vi "Read Configuration with Unknown Modules.vi"() -> ()   [LabVIEW 2017]
uses:
  Types/Module Channel Settings.ctl
  <vilib>/addons/VeriStand Custom Device Scripting APIs/Scan Engine/Modules/Mode Classes/Controls/counter driven output channel settings.ctl
  <vilib>/addons/VeriStand Custom Device Scripting APIs/Scan Engine/Modules/Channel Classes/Counter Driven Output Channel/Counter Driven State.ctl
  <vilib>/addons/VeriStand Custom Device Scripting APIs/Scan Engine/Modules/Mode Classes/Controls/pwm channel settings.ctl
  <vilib>/addons/VeriStand Custom Device Scripting APIs/Scan Engine/Modules/Channel Classes/PWM Output Channel/Frequency.ctl
  <vilib>/addons/VeriStand Custom Device Scripting APIs/Scan Engine/Modules/NI 9474/NI 9474.lvclass
  f6bbfe02-b953-4ef2-a52c-5a4fac125821.vi
  <vilib>/addons/VeriStand Custom Device Scripting APIs/Scan Engine/Scan Engine Dependencies.llb/Set Error.vi
  <vilib>/Utility/error.llb/Clear Errors.vi
  <vilib>/addons/VeriStand Custom Device Scripting APIs/Scan Engine/Utility/Convert Slot Configuration to 9212.vi
  <vilib>/addons/VeriStand Custom Device Scripting APIs/Scan Engine/Utility/Convert Slot Configuration to 9213.vi
  <vilib>/addons/VeriStand Custom Device Scripting APIs/Scan Engine/Modules.lvlibp/SD Module/SD Module.lvclass
  C:/Program Files (x86)/National Instruments/LabVIEW 2017/vi.lib/addons/VeriStand Custom Device Scripting APIs/Scan Engine/Modules.lvlibp/RSI Module/RSI Module.lvclass
  <vilib>/addons/VeriStand Custom Device Scripting APIs/Scan Engine/Modules/NI 9212/NI 9212.lvclass
  C:/Program Files (x86)/National Instruments/LabVIEW 2017/vi.lib/addons/VeriStand Custom Device Scripting APIs/Scan Engine/Modules/Module/Module.lvclass
  <vilib>/addons/VeriStand Custom Device Scripting APIs/Scan Engine/Modules/NI 9213/NI 9213.lvclass
  <vilib>/addons/VeriStand Custom Device Scripting APIs/Scan Engine/Modules/NI 9224/NI 9224.lvclass
  <vilib>/addons/VeriStand Custom Device Scripting APIs/Scan Engine/Modules/NI 9228/NI 9228.lvclass
  <vilib>/addons/VeriStand Custom Device Scripting APIs/Scan Engine/Modules.lvlibp/RSI Module/Read Module Page Property.vi
  <vilib>/addons/VeriStand Custom Device Scripting APIs/Scan Engine/Modules.lvlibp/RSI Module/Read Model.vi
  <vilib>/addons/VeriStand Custom Device Scripting APIs/Scan Engine/Utility/Convert Module Model to Module Class.vi
  <vilib>/addons/VeriStand Custom Device Scripting APIs/Scan Engine/Modules.lvlibp/SD Module/Read DIO mode.vi
  <vilib>/addons/VeriStand Custom Device Scripting APIs/Scan Engine/Modules.lvlibp/RSI Module/Read Channels.vi
  <vilib>/addons/VeriStand Custom Device Scripting APIs/Scan Engine/Utility/Convert to DI Module.vi
  <vilib>/addons/VeriStand Custom Device Scripting APIs/Scan Engine/Utility/Convert to DO Module.vi
  <vilib>/addons/VeriStand Custom Device Scripting APIs/Scan Engine/Utility/Convert to CI PWM Module.vi
  <vilib>/addons/VeriStand Custom Device Scripting APIs/Scan Engine/Utility/Convert to CDO Module.vi
  <vilib>/addons/VeriStand Custom Device Scripting APIs/Scan Engine/Utility/Convert to PWM Module.vi
  <vilib>/addons/VeriStand Custom Device Scripting APIs/Scan Engine/Scan Engine Dependencies.llb/Error Strings.vi
  <vilib>/addons/VeriStand Custom Device Scripting APIs/Scan Engine/Utility/Get Channel Names and Default Values for Slot.vi
  <vilib>/addons/VeriStand Custom Device Scripting APIs/Scan Engine/Modules/NI 9212/Create NI 9212.vi
  <vilib>/addons/VeriStand Custom Device Scripting APIs/Scan Engine/Modules/NI 9213/Create NI 9213.vi
  <vilib>/addons/VeriStand Custom Device Scripting APIs/Scan Engine/Utility/Convert to AI Module.vi
  <vilib>/addons/VeriStand Custom Device Scripting APIs/Scan Engine/Utility/Convert to AI Vrms Module.vi
  <vilib>/addons/VeriStand Custom Device Scripting APIs/Scan Engine/Utility/Convert to AI Arms Module.vi
  <vilib>/addons/VeriStand Custom Device Scripting APIs/Scan Engine/Utility/Convert to DIO Module.vi
  <vilib>/addons/VeriStand Custom Device Scripting APIs/Scan Engine/Modules/NI 9474/Read NI 9474 - Counter Driven Output.vi
  <vilib>/addons/VeriStand Custom Device Scripting APIs/Scan Engine/Modules/NI 9474/Read NI 9474 - PWM Output.vi
  <vilib>/addons/VeriStand Custom Device Scripting APIs/Scan Engine/Modules/Module/Module.lvclass
  <vilib>/addons/VeriStand Custom Device Scripting APIs/Scan Engine/Modules.lvlibp/9212/9212.lvclass
  <vilib>/addons/VeriStand Custom Device Scripting APIs/Scan Engine/Modules.lvlibp/9213/9213.lvclass
  <vilib>/addons/VeriStand Custom Device Scripting APIs/Scan Engine/Modules.lvlibp/9224/9224.lvclass
  SubVIs/Scan Engine Example Support.lvlib
  <vilib>/addons/VeriStand Custom Device Scripting APIs/Scan Engine/Scan Engine Scripting.lvlib
  <vilib>/addons/VeriStand Custom Device Scripting APIs/Scan Engine/Modules/Channel Classes/PWM Output Channel/PWM Output Channel.lvclass
  <vilib>/addons/VeriStand Custom Device Scripting APIs/Scan Engine/Modules/Channel Classes/Counter Driven Output Channel/Counter Driven Output Channel.lvclass
panel:
  out "Channel Settings":T1[](array[typedef])
  # "Overview: Demonstrates using the Scan Engine and EtherCAT scripting API to read a configuration from a system definition file that contains a Scan Engine Custom Device.\n\nInstructions:\nRun the VI."
  # "Slot Properties"
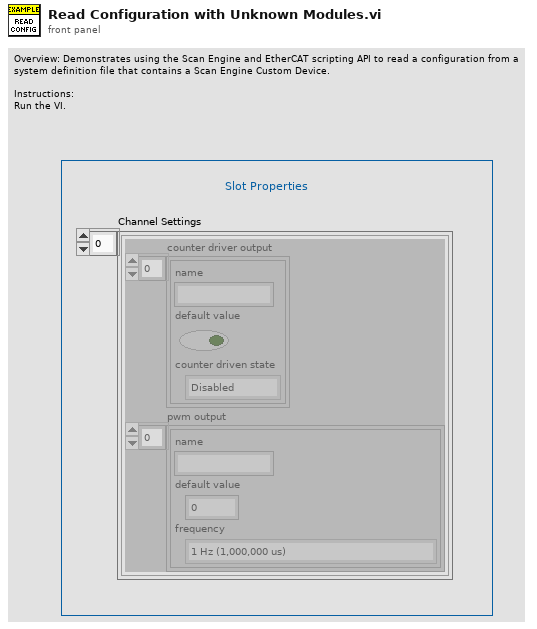
[diagram p1: front panel]
types:
  T1 = typedef "Module Channel Settings.ctl" = cluster{"counter driver output":T2[], "pwm output":T4[]}
  T2 = typedef "Scan Engine Scripting.lvlib/counter driven output channel settings.ctl" = cluster{"name":string, "default value":bool, "counter driven state":T3}
  T3 = typedef "Scan Engine Scripting.lvlib/Counter Driven Output Channel.lvclass/Counter Driven State.ctl" = enum16{"Disabled", "Enabled"}
  T4 = typedef "Scan Engine Scripting.lvlib/pwm channel settings.ctl" = cluster{"name":string, "default value":dbl, "frequency":T5}
  T5 = typedef "Scan Engine Scripting.lvlib/PWM Output Channel.lvclass/Frequency.ctl" = enum16{"1 Hz (1,000,000 us)", "50 Hz (20,000 us)", "250 Hz (4,000 us)", "500 Hz (2,000 us)", "1 kHz (1,000 us)", "5 kHz (200 us)", "10 kHz (100 us)", "20 kHz (50 us)"}
  T6 = typedef "Custom Device API.lvlib/Custom Device Item Ref.ctl" = u64
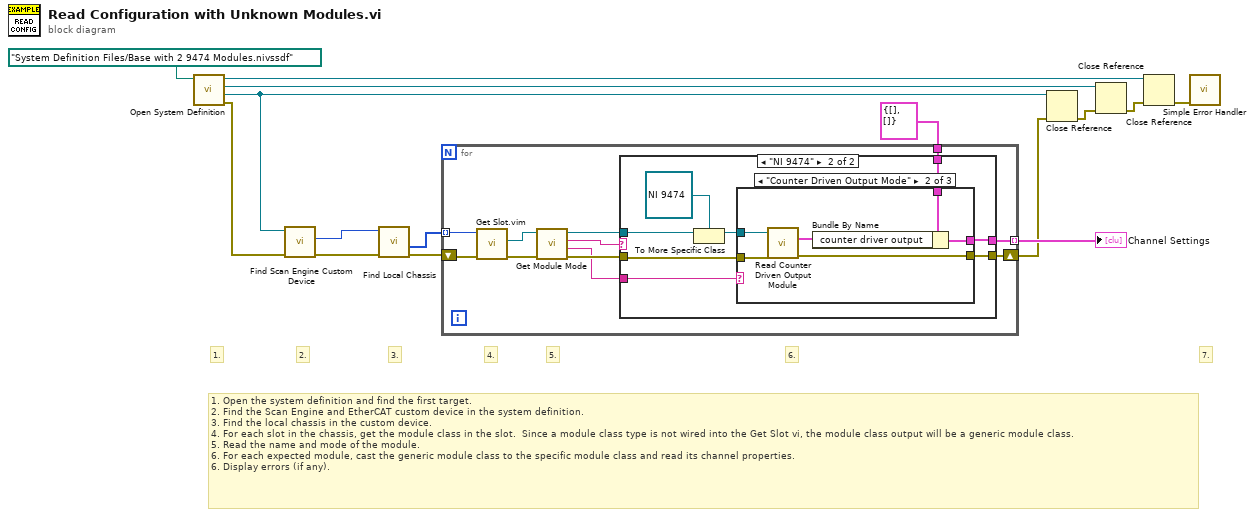
[diagram p0: block diagram]
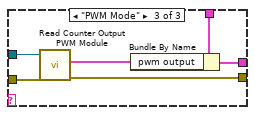
[diagram p4: hidden frame]
diagram:
  # "6."
  # "5."
  # "4."
  # "3."
  # "2."
  # "7."
  # "1."
  # "1. Open the system definition and find the first target.\n2. Find the Scan Engine and EtherCAT custom device in the system definition.\n3. Find the local chassis in the custom device.\n4. For each slot in the chassis, get the module class in the slot.  Since a module class type is not wired into the Get Slot vi, the module class output will be a generic module class.\n5. Read the name and mode of the module.\n6. For each expected module, cast the generic module class to the specific module class and read its channel properties.\n6. Display errors (if any)."
  n1 = call "Open System Definition.vi"("System Definition File"=path "System Definition Files/Base with 2 9474 Modules.nivssdf" ("Input System Definition File")) -> ("error out"=w6:errorcluster, "Target Refnum"=w4:refnum<k24>, "Root Refnum"=w8:refnum<k24>, "System Definition Refnum"=w9:refnum<k24>)  [unwired: 7 in]
  n2 = call <vilib>:"Find Scan Engine Custom Device.vi"("error in"=w6, "target in"=w4) -> ("error out"=w7:errorcluster, "scan engine custom device ref"=w10:T6)  [unwired: 6 in, 2 out]
  n3 = call <vilib>:"Find Local Chassis.vi"("error in"=w7, "scan engine custom device ref in"=w10) -> ("error out"=w2:errorcluster, "slots refs"=w11:T6[])  [unwired: 4 in, 4 out]
  n4 = for {
    tunnel: [w22] -> w5 mode=indexing
    tunnel: w11 -> [w26] mode=indexing
    shift-right: [w25] -> w3
    shift-left: w2 -> [w24]
    tunnel: T1 {"counter driver output"=[], "pwm output"=[]} ("Cluster") -> [w23]
    n5 = call "Get Slot.vim"("error in"=w24, "slot ref in"=w26) -> ("error out"=w21:errorcluster, "module"=w20:refnum<class "Module.lvclass">)  [unwired: 6 in, 2 out]
    n6 = call "Get Module Mode.vi"("error in (no error)"=w21, "module in"=w20) -> ("error out"=w18:errorcluster, "module mode"=w16:string, "module name"=w17:string, "module out"=w19:refnum<class "Module.lvclass">)  [unwired: 6 in]
    n7 = case shown="\"NI 9474\"" w17 {
      tunnel: [_ w35] -> w22
      tunnel: w18 -> [w27 w32]
      tunnel: [w27 w31] -> w25
      tunnel: w23 -> [_ w30]
      tunnel: w19 -> [_ w28]
      tunnel: w16 -> [_ w29]
      frame Default {
        # "Note: Add additional cases for each supported type"
      }
      frame "NI 9474" {
        n8 = To More Specific Class(target class=refnum<class "NI 9474.lvclass"> refnum ("NI 9474 in"), reference=w28) -> (specific class reference=w33:refnum<class "NI 9474.lvclass">)  [unwired: 1 in, 1 out]
        n9 = case shown="\"Counter Driven Output Mode\"" w29 {
          tunnel: [_ w38 w43] -> w35
          tunnel: w33 -> [_ w42 w48]
          tunnel: w32 -> [w36 w41 w47]
          tunnel: [w36 w40 w46] -> w31
          tunnel: w30 -> [_ w39 w45]
          frame Default {
          }
          frame "Counter Driven Output Mode" {
            n10 = call-poly <vilib>:"Read Counter Driven Output Module.vi"("error in"=w41, "NI 9474 in"=w42) -> ("error out"=w40:errorcluster, "channel settings"=w37:T2[])  [unwired: 6 in, 2 out]
            n11 = Bundle By Name(cluster=w39, "counter driver output"=w37) -> (w38:T1)
          }
          frame "PWM Mode" {
            n12 = call-poly <vilib>:"Read Counter Output PWM Module.vi"("error in"=w47, "NI 9474 in"=w48) -> ("error out"=w46:errorcluster, "channel settings"=w44:T4[])  [unwired: 7 in, 1 out]
            n13 = Bundle By Name(cluster=w45, "pwm output"=w44) -> (w43:T1)
          }
        }
      }
    }
  }
  "Channel Settings" <- w5
  n14 = Close Reference(reference=w4, error in (no error)=w3) -> (error out=w14:errorcluster)
  n15 = Close Reference(reference=w8, error in (no error)=w14) -> (error out=w15:errorcluster)
  n16 = Close Reference(reference=w9, error in (no error)=w15) -> (error out=w13:errorcluster)
  n17 = call <vilib>:"Simple Error Handler.vi"("error in (no error)"=w13) -> ()  [unwired: 1 in, 8 out]
